vi "Setup DPMs.vi"(8 "Error in":errorcluster caption="Error in (no error)", 10 "DPMs":refnum<class "Instrument.lvclass">[](array[class]), 11 "Test Class in":refnum<class "Test Class.lvclass">) -> (0 "Error out":errorcluster)   [LabVIEW 2015, in "Instrument Setup.lvclass"]
uses:
  Instrument Setup.lvclass
  Classes/Instruments/Instrument/Class/Instrument.lvclass
  Test Class/Test Class.lvclass
  Classes/Instruments/Digital Power Meter/Digital Power Meter/Class/Digital Power Meter.lvclass
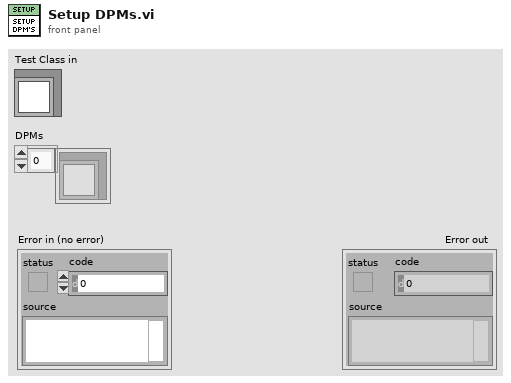
[diagram p1: front panel]
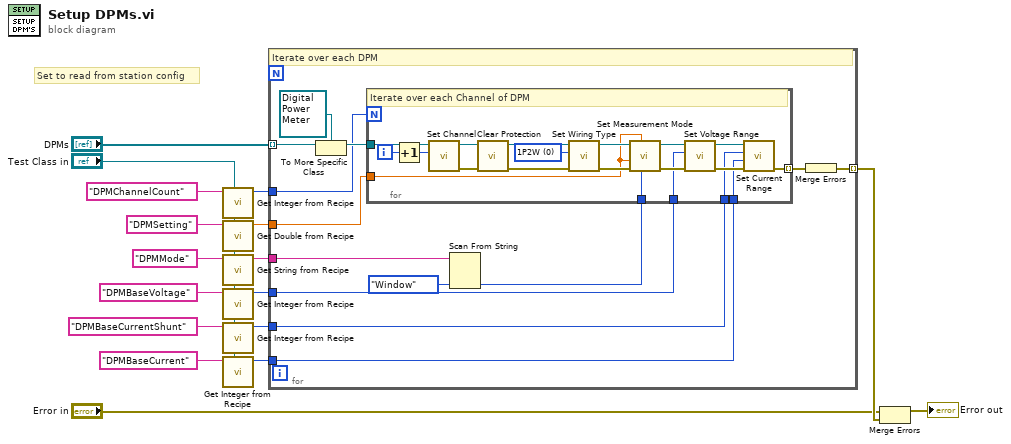
[diagram p0: block diagram]
diagram:
  # "Set to read from station config"
  n1 = call "Get Integer from Recipe.vi"("Test Class in"="Test Class in", "Name"="DPMChannelCount") -> ("Value"=w2:i32)  [unwired: 7 in, 2 out]
  n2 = call "Get Double from Recipe.vi"("Test Class in"="Test Class in", "Name"="DPMSetting") -> ("Value"=w14:dbl)  [unwired: 7 in, 2 out]
  n3 = call "Get String from Recipe.vi"("Test Class in"="Test Class in", "Name"="DPMMode") -> ("Value"=w5:string)  [unwired: 7 in, 2 out]
  n4 = call "Get Integer from Recipe.vi"("Test Class in"="Test Class in", "Name"="DPMBaseVoltage") -> ("Value"=w6:i32)  [unwired: 7 in, 2 out]
  n5 = call "Get Integer from Recipe.vi"("Test Class in"="Test Class in", "Name"="DPMBaseCurrentShunt") -> ("Value"=w7:i32)  [unwired: 7 in, 2 out]
  n6 = call "Get Integer from Recipe.vi"("Test Class in"="Test Class in", "Name"="DPMBaseCurrent") -> ("Value"=w8:i32)  [unwired: 7 in, 2 out]
  n7 = for {
    tunnel: "DPMs" -> [w23] mode=indexing
    tunnel: w14 -> [w29]
    tunnel: [w28] -> w16 mode=indexing
    tunnel: w5 -> [w27]
    tunnel: w6 -> [w21]
    tunnel: w7 -> [w20]
    tunnel: w8 -> [w19]
    tunnel: w2 -> [w18]
    # "Iterate over each DPM"
    n8 = To More Specific Class(target class=refnum<class "Digital Power Meter.lvclass"> refnum ("Digital Power Meter.lvlib:Digital Power Meter.lvclass"), reference=w23) -> (specific class reference=w22:refnum<class "Digital Power Meter.lvclass">)  [unwired: 1 in, 1 out]
    n9 = Scan From String(input string=w27, default 1=enum16{"Window", "Average"}."Window" ("Measurement Mode")) -> (output 1=w25:enum16{"Window", "Average"})  [unwired: 3 in, 3 out]
    n10 = for {
      N: w18 -> [_]
      tunnel: w22 -> [w50]
      tunnel: [w34] -> w30 mode=indexing
      tunnel: w29 -> [w40]
      tunnel: w25 -> [w39]
      tunnel: w21 -> [w33]
      tunnel: w20 -> [w32]
      tunnel: w19 -> [w31]
      i -> [w49]
      w44 = 0 items=["1P2W", "1P3W", "3P3W", "3P4W"] ("Input Wiring Type")
      # "Iterate over each Channel of DPM"
      n11 = Increment(x=w49) -> (x+1=w48:i32)
      n12 = call-dynamic "Set Channel.vi"("Channel"=w48, "Acrobat Template in"=w50) -> ("error out"=w46:errorcluster, "Acrobat Template out"=w47:refnum<class "Digital Power Meter.lvclass">)  [unwired: 8 in]
      n13 = call-dynamic "Clear Protection.vi"("error in (no error)"=w46, "Acrobat Template in"=w47) -> ("error out"=w43:errorcluster, "Acrobat Template out"=w45:refnum<class "Digital Power Meter.lvclass">)  [unwired: 8 in]
      n14 = call-dynamic "Set Wiring Type.vi"("error in (no error)"=w43, "Input Wiring Type"=w44, "Acrobat Template in"=w45) -> ("error out"=w41:errorcluster, "Acrobat Template out"=w42:refnum<class "Digital Power Meter.lvclass">)  [unwired: 7 in]
      n15 = call-dynamic "Set Measurement Mode.vi"("Measurement Mode"=w39, "Num of Averages"=w40, "error in (no error)"=w41, "Window Size (sec)"=w40, "Acrobat Template in"=w42) -> ("error out"=w36:errorcluster, "Acrobat Template out"=w38:refnum<class "Digital Power Meter.lvclass">)  [unwired: 5 in]
      n16 = call-dynamic "Set Voltage Range.vi"("error in (no error)"=w36, "Voltage Range"=w33, "Acrobat Template in"=w38) -> ("error out"=w35:errorcluster, "Acrobat Template out"=w37:refnum<class "Digital Power Meter.lvclass">)  [unwired: 7 in]
      n17 = call-dynamic "Set Current Range.vi"("error in (no error)"=w35, "Current Range In"=w31, "Shunt Range In"=w32, "Acrobat Template in"=w37) -> ("error out"=w34:errorcluster)  [unwired: 6 in, 1 out]
    }
    n18 = Merge Errors(w30) -> (w28:errorcluster)
  }
  n19 = Merge Errors("Error in", w16) -> (→"Error out":errorcluster)
